vi "fromStringImage.vi"(1 "value":string[][](array[string]), 2 "attribute name":string, 3 "device name":string) -> (0 "attribute value":T1={"device name"="", "attribute name"="", "quality value"=enum."VALID", "quality string"="", "timestamp"=0.0, "dim. x"=0, "dim. y"=0, "value"=[], "error code"=0, "error stack"=[], "data type"=enum."STRING_SPE"})   [LabVIEW 2014, in "tango.lvlib"]
uses:
  tango.lvlib
  Common VIs/Typedefs/_AttributeValue_t.ctl
  Common VIs/Typedefs/_AttributeQuality_t.ctl
  Common VIs/Typedefs/_AttributeDataType_t.ctl
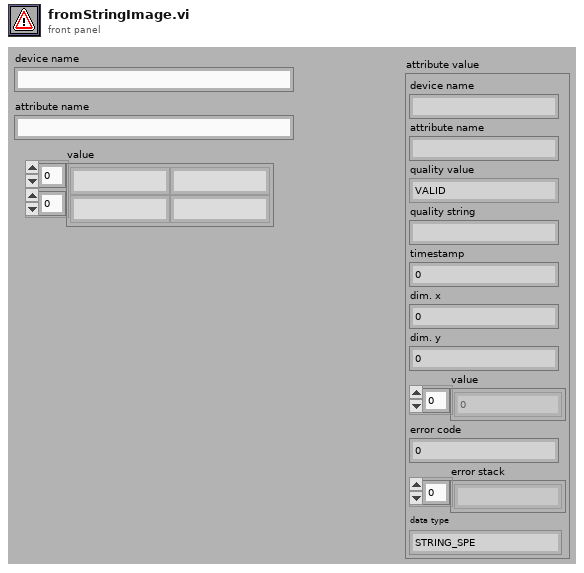
[diagram p1: front panel]
types:
  T1 = typedef "tango.lvlib/_AttributeValue_t.ctl" = cluster{"device name":string, "attribute name":string, "quality value":T2, "quality string":string, "timestamp":dbl, "dim. x":i32, "dim. y":i32, "value":u8[], "error code":i32, "error stack":string[], "data type":T3}
  T2 = typedef "tango.lvlib/_AttributeQuality_t.ctl" = enum16{"VALID", "INVALID", "ALARM", "CHANGING", "UNKNOWN_QUALITY"}
  T3 = typedef "tango.lvlib/_AttributeDataType_t.ctl" = enum16{"STATE_SCA", "STATE_SPE", "STATE_IMG", "STRING_SCA", "STRING_SPE", "STRING_IMG", "BOOL_SCA", "BOOL_SPE", "BOOL_IMG", "UCHAR_SCA", "UCHAR_SPE", "UCHAR_IMG", "SHORT_SCA", "SHORT_SPE", "SHORT_IMG", "USHORT_SCA", "USHORT_SPE", "USHORT_IMG", "LONG_SCA", "LONG_SPE", "LONG_IMG", "ULONG_SCA", "ULONG_SPE", "ULONG_IMG", "LONG64_SCA", "LONG64_SPE", "LONG64_IMG", "ULONG64_SCA", "ULONG64_SPE", "ULONG64_IMG", "FLOAT_SCA", "FLOAT_SPE", "FLOAT_IMG", "DOUBLE_SCA", "DOUBLE_SPE", "DOUBLE_IMG", "UNKNOWN_DATA_TYPE"}
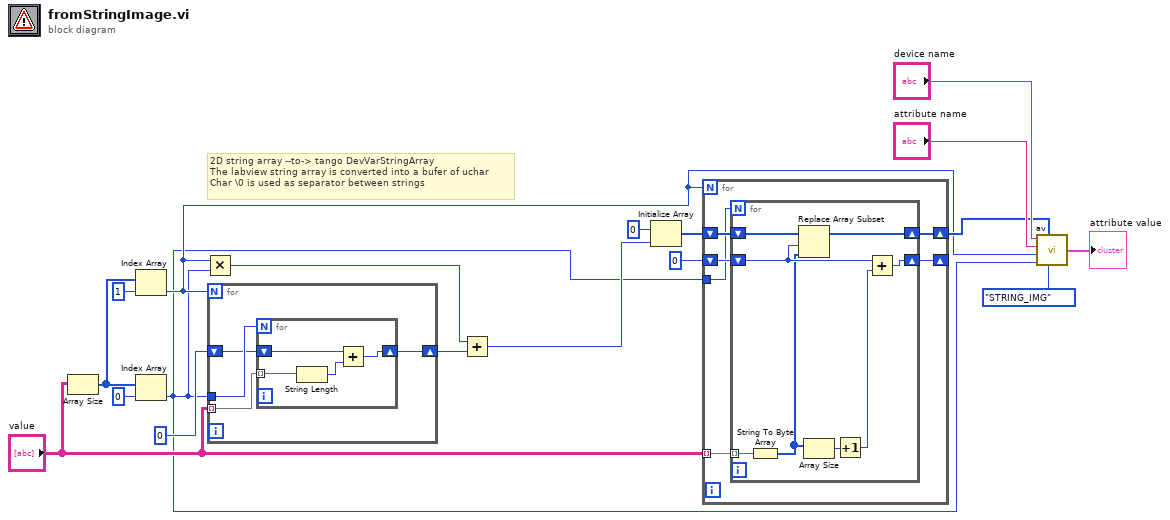
[diagram p0: block diagram]
diagram:
  # "2D string array --to-> tango DevVarStringArray\nThe labview string array is converted into a bufer of uchar\nChar \\0 is used as separator between strings"
  n1 = Array Size(array="value") -> (size(s)=w13:i32[])
  n2 = Index Array(array=w13, index=1) -> (element=w4:i32)
  n3 = Index Array(array=w13, index=0) -> (element=w2:i32)
  n4 = Multiply(x=w4, y=w2) -> (x*y=w7:i32)
  n5 = for {
    N: w4 -> [_]
    tunnel: w2 -> [w22]
    tunnel: "value" -> [w21] mode=indexing
    shift-right: [w19] -> w9
    shift-left: 0 -> [w20]
    n6 = for {
      N: w22 -> [_]
      tunnel: w21 -> [w26] mode=indexing
      shift-right: [w24] -> w19
      shift-left: w20 -> [w23]
      n7 = String Length(string=w26) -> (length=w25:i32)
      n8 = Add(x=w23, y=w25) -> (x+y=w24:i32)
    }
  }
  n9 = Add(x=w7, y=w9) -> (x+y=w6:i32)
  n10 = Initialize Array(u8 0, w6) -> (w11:u8[])
  n11 = for {
    N: w4 -> [_]
    tunnel: w2 -> [w30]
    tunnel: "value" -> [w29] mode=indexing
    shift-right: [w27] -> _
    shift-left: 0 -> [w31]
    shift-right: [w28] -> w8
    shift-left: w11 -> [w32]
    n12 = for {
      N: w30 -> [_]
      shift-right: [w39] -> w28
      shift-left: w32 -> [w40]
      shift-right: [w37] -> w27
      shift-left: w31 -> [w35]
      tunnel: w29 -> [w34] mode=indexing
      n13 = String To Byte Array(string=w34) -> (unsigned byte array=w33:u8[])
      n14 = Replace Array Subset(array=w40, new element=w33, index=w35) -> (w39:u8[])
      n15 = Array Size(array=w33) -> (size(s)=w38:i32)
      n16 = Increment(x=w38) -> (x+1=w36:i32)
      n17 = Add(x=w35, y=w36) -> (x+y=w37:i32)
    }
  }
  n18 = call "av.vi"("tango data type"=_AttributeDataType_t."STRING_IMG", "data"=w8, "dim. y"=w2, "dim. x"=w4, "attribute name"="attribute name", "device name"="device name") -> ("attribute value"=→"attribute value":T1)
